vi "ep_Check Input Size (1 Motor).vi"(7 "check? (F)":bool, 8 "error in (no error)":errorcluster, 10 "algorithm":T1=enum."3-phase signals", 11 "number of channels":i32) -> (0 "error out":errorcluster)   [LabVIEW 2014, in "NI_EP_Motor Monitoring.lvlib"]
uses:
  <vilib>/addons/Electrical Power/Motor Monitoring/NI_EP_Motor Monitoring.lvlib
  <vilib>/addons/Electrical Power/Motor Monitoring/subVIs/ep_Demodulation Algorithm.ctl
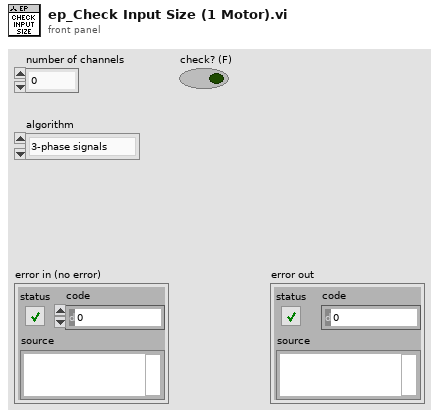
[diagram p1: front panel]
types:
  T1 = typedef "NI_EP_Motor Monitoring.lvlib/ep_Demodulation Algorithm.ctl" = enum16{"1-phase signal", "3-phase signals"}
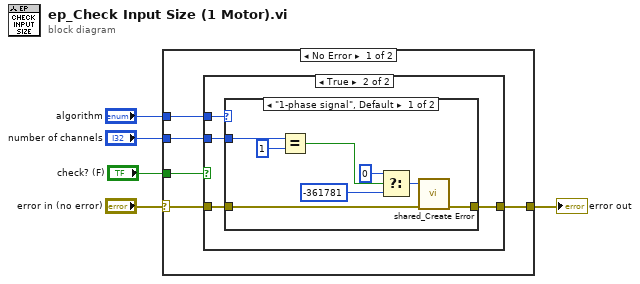
[diagram p0: block diagram]
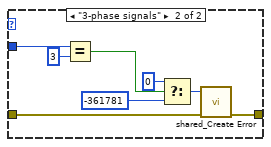
[diagram p3: hidden frame]
diagram:
  n1 = case shown="No Error" "error in (no error)" {
    selector: "error in (no error)" -> [w7 w32]
    tunnel: "number of channels" -> [w8 _]
    tunnel: "algorithm" -> [w9 _]
    tunnel: [w10 w32] -> w2
    tunnel: "check? (F)" -> [w6 _]
    frame No Error {
      n2 = case shown="True" w6 {
        tunnel: [w11 w15] -> w10
        tunnel: w9 -> [_ w14]
        tunnel: w8 -> [_ w13]
        tunnel: w7 -> [w11 w12]
        frame False {
        }
        frame True {
          n3 = case shown="\"1-phase signal\", Default" w14 {
            tunnel: w13 -> [w17 w25]
            tunnel: w12 -> [w19 w26]
            tunnel: [w18 w27] -> w15
            frame "1-phase signal", Default {
              n4 = Equal?(x=w17, y=1) -> (x = y?=w20:bool)
              n5 = Select(t=0 ("y"), s=w20, f=-361781 ("y")) -> (s? t:f=w21:i32)
              n6 = call <vilib>:"shared_Create Error.vi"("error in (no error)"=w19, "error code (0)"=w21) -> ("error out"=w18:errorcluster)  [unwired: 9 in]
            }
            frame "3-phase signals" {
              n7 = Equal?(x=w25, y=3) -> (x = y?=w24:bool)
              n8 = Select(t=0 ("y"), s=w24, f=-361781 ("y")) -> (s? t:f=w28:i32)
              n9 = call <vilib>:"shared_Create Error.vi"("error in (no error)"=w26, "error code (0)"=w28) -> ("error out"=w27:errorcluster)  [unwired: 9 in]
            }
          }
        }
      }
    }
    frame Error {
    }
  }
  "error out" <- w2
